vi "UDP_send_002.vi"() -> ()   [LabVIEW 2019]
panel:
  in  "Message":string="Hello!"
  in  "stop":bool
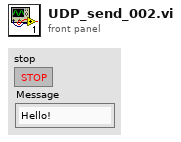
[diagram p1: front panel]
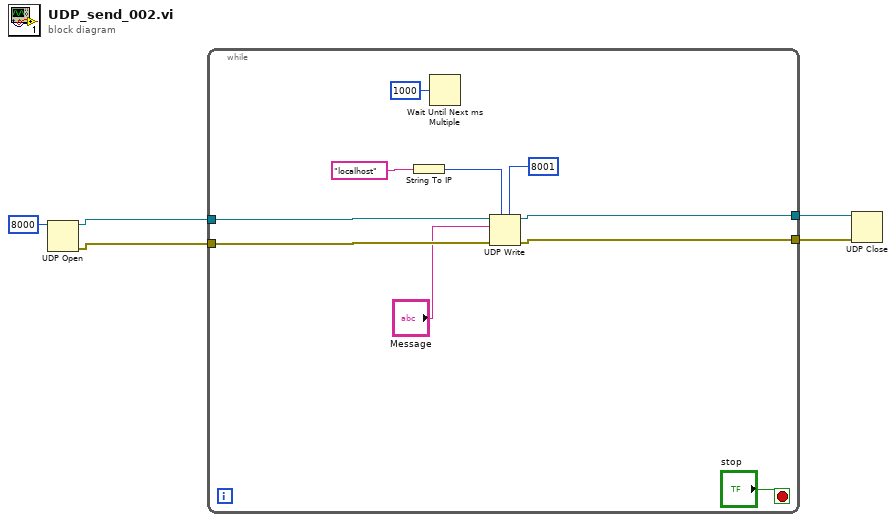
[diagram p0: block diagram]
diagram:
  n1 = UDP Open(11:u16 8000 ("port")) -> (port=w3:refnum<k16>, 0:w5:errorcluster)  [unwired: 4 in, 1 out]
  n2 = while {
    tunnel: w5 -> [w14]
    tunnel: [w13] -> w4
    tunnel: w3 -> [w12]
    tunnel: [w11] -> w2
    stop <- "stop" stop-if-true
    n3 = String To IP(1:"localhost") -> (0:w7:u32)
    n4 = Wait Until Next ms Multiple(millisecond multiple=u32 1000) -> ()  [unwired: 1 out]
    n5 = UDP Write(address=w7, port or service name=u16 8001, connection ID=w12, data in="Message", 8:w14) -> (error out=w13:errorcluster, 3:w11:refnum<k16>)  [unwired: 1 in]
  }
  n6 = UDP Close(connection ID=w2, 8:w4) -> ()  [unwired: 2 out]
